vi "Decompress String.vi"(8 "error in (no error)":errorcluster, 10 "Compressed String":string) -> (0 "error out":errorcluster, 2 "Decompressed String":string)   [LabVIEW 2018, in "Kompress.lvlib"]
uses:
  Kompress.lvlib
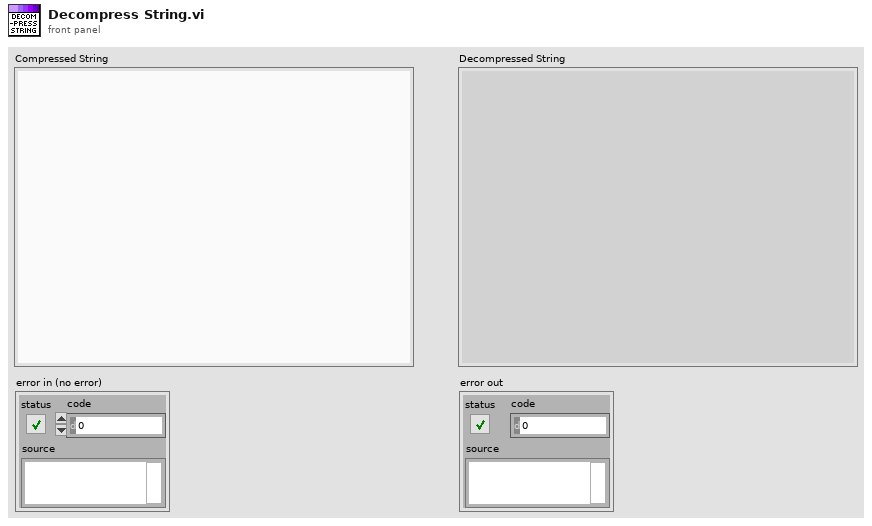
[diagram p1: front panel]
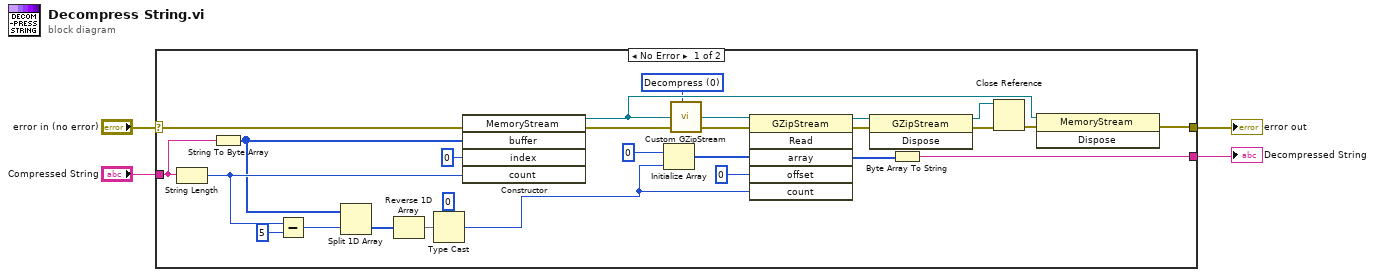
[diagram p0: block diagram]
diagram:
  n1 = case shown="No Error" "error in (no error)" {
    selector: "error in (no error)" -> [w16 w32]
    tunnel: [w18 _] -> w4
    tunnel: [w10 w32] -> w3
    tunnel: "Compressed String" -> [w17 _]
    frame No Error {
      w5 = 0 items=["Decompress", "Compress"] ("CompressionMode")
      n2 = String Length(string=w17) -> (length=w20:i32)
      n3 = String To Byte Array(string=w17) -> (unsigned byte array=w19:u8[])
      n4 = Subtract(x=w20, y=5) -> (x-y=w30:i32)
      n5 = Split 1D Array(array=w19, index=w30) -> (second subarray=w29:u8[])  [unwired: 1 out]
      n6 = Reverse 1D Array(array=w29) -> (reversed array=w21:u8[])
      n7 = Type Cast(type=u32 0, x=w21) -> (*(type *) &x=w23:u32)
      n8 = constructor class="MemoryStream" ("mso")(error in=w16, "buffer"=w19, "index"=0, "count"=w20) -> (reference out=w8:refnum<k24>, error out=w9:errorcluster)  [unwired: 2 in, 4 out]
      n9 = Initialize Array(u8 0 ("offset"), w23) -> (w24:u8[])
      n10 = call "Custom GZipStream.vi"("Compression Mode"=w5, "System.IO.Stream"=w8, "error in (no error)"=w9) -> ("System.IO.Compression.GZipStream"=w7:refnum<k24>, "error out"=w6:errorcluster)  [unwired: 3 in]
      n11 = invoke class="GZipStream" method="Read"(reference=w7, error in=w6, "array"=w24, "offset"=0, "count"=w23) -> (reference out=w13:refnum<k24>, error out=w14:errorcluster, "array"=w22:u8[])  [unwired: 1 in, 3 out]
      n12 = invoke class="GZipStream" method="Dispose"(reference=w13, error in=w14) -> (reference out=w12:refnum<k24>, error out=w15:errorcluster)  [unwired: 1 in, 1 out]
      n13 = Byte Array To String(unsigned byte array=w22) -> (string=w18:string)
      n14 = Close Reference(reference=w12, error in (no error)=w15) -> (error out=w11:errorcluster)
      n15 = invoke class="MemoryStream" method="Dispose"(reference=w8, error in=w11) -> (error out=w10:errorcluster)  [unwired: 1 in, 2 out]
    }
    frame Error {
    }
  }
  "Decompressed String" <- w4
  "error out" <- w3
